vi "Check Camera Settings.vi"(11 "Camera Settings In":T1={"Exposure Time (ms)"=100.0, "Binning"=enum."2x2", "Scan Mode"=0, "Frames to Acquire"=1000.0, "Pixel Correction"=FALSE, "Frames to Skip"=0, "File Path"=path "", "Duty cycle"=0.0, "ALEX"=FALSE, "Shutter Enable"=[], "fluidics trigger, ms (0=disabled)"=0.0, "Bit Depth"=16, "Image Width (px)"=0, "Image Height (px)"=0, "Horizontal Offset (px)"=0, "Vertical Offset (px)"=0} {"fluidics trigger, ms (0=disabled)" max=60000.0 step=1.0; "Exposure Time (ms)" min=1.0 max=10000.0 step=1.0}) -> (1 "Ok":bool)   [LabVIEW 2023]
uses:
  Type Defs/Camera Settings.ctl
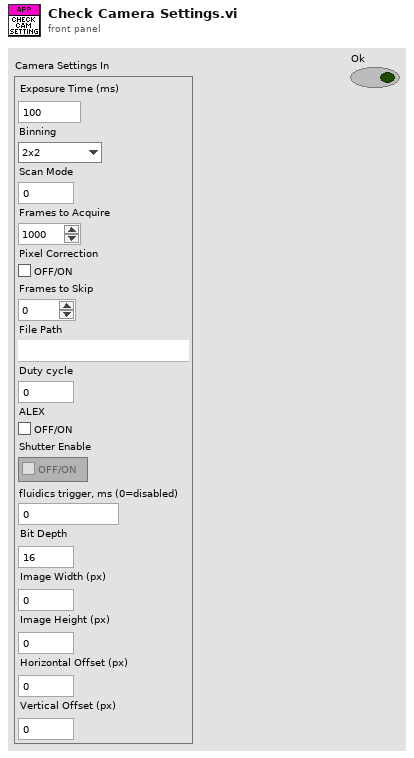
[diagram p1: front panel]
types:
  T1 = typedef "Camera Settings.ctl" = cluster{"Exposure Time (ms)":dbl, "Binning":enum16{"1x1", "2x2", "4x4"}, "Scan Mode":i32, "Frames to Acquire":dbl, "Pixel Correction":bool, "Frames to Skip":u32, "File Path":path, "Duty cycle":dbl, "ALEX":bool, "Shutter Enable":bool[], "fluidics trigger, ms (0=disabled)":dbl, "Bit Depth":u16, "Image Width (px)":u16, "Image Height (px)":u16, "Horizontal Offset (px)":u16, "Vertical Offset (px)":u16}
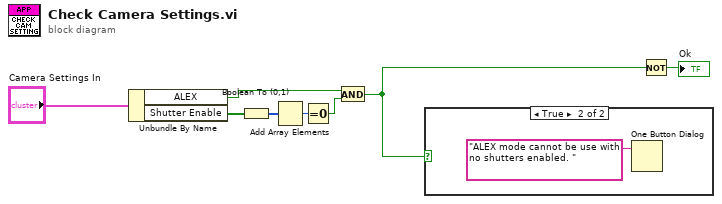
[diagram p0: block diagram]
diagram:
  n1 = Unbundle By Name("Camera Settings In") -> ("ALEX"=w6:bool, "Shutter Enable"=w7:bool[])
  n2 = Boolean To (0,1)(Boolean=w7) -> (0, 1=w8:i16[])
  n3 = Add Array Elements(numeric array=w8) -> (sum=w5:i16)
  n4 = Equal To 0?(x=w5) -> (x = 0?=w4:bool)
  n5 = And(x=w6, y=w4) -> (x .and. y?=w1:bool)
  n6 = case shown="True" w1 {
    frame False {
    }
    frame True {
      n7 = One Button Dialog(message="ALEX mode cannot be use with no shutters enabled. ") -> ()  [unwired: 1 in, 1 out]
    }
  }
  n8 = Not(x=w1) -> (.not. x?=→"Ok":bool)
